vi "Login-Window.vi"(8 "Error in":errorcluster caption="Error in (no error)", 11 "Options":T1={"HideMain(T)"=TRUE, "RetryAllowed(T)"=TRUE, "LastUserToINI(T)"=TRUE}) -> (0 "Error out":errorcluster={"status"=TRUE, "code"=43, "source"="Operation cancelled by user."}, 1 "Valid User":bool, 3 "User Info":T3={"UserName"="", "Password"="", "Role"=enum."Admin"})   [LabVIEW 2017, in "Login-UI.lvlib"]
uses:
  Login-UI.lvlib
  _Typedef/Login-Account.ctl
  _Typedef/Login-Password.ctl
  _Typedef/Login-Admin.ctl
  _Typedef/Login-Confirm.ctl
  _Typedef/User-Info.ctl
  _Typedef/User-Role.ctl
  _Support/_password_db_oper.ctl
  82dbac5f-f66d-497b-81a9-0f95a8baf484.vi
  <resource>/dialog/lvconfig.llb/LV Config Read String.vi
  <resource>/dialog/lvconfig.llb/LV Config Write String.vi
panel:
  in  "UserManage":T2
  in  "Login":T5
  in  "Password":T6
  in  "UserName":T7
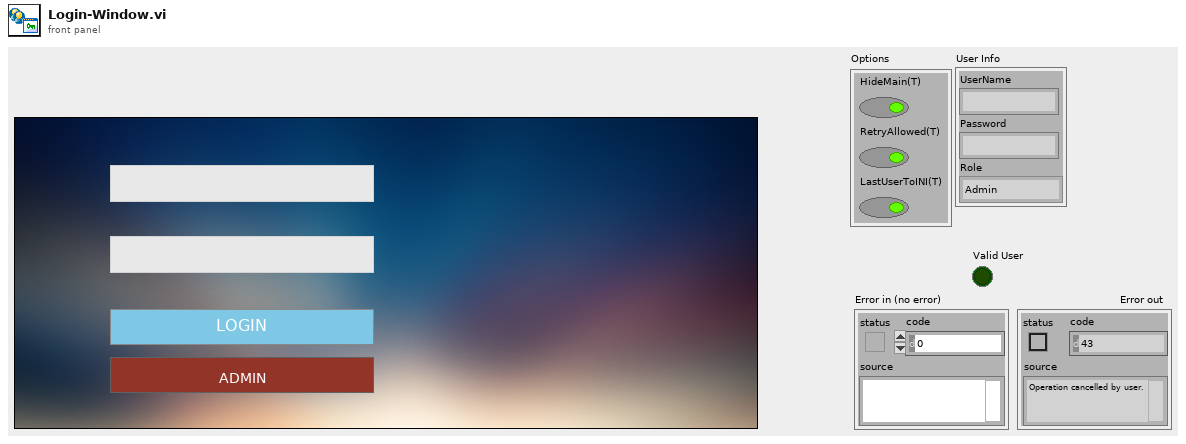
[diagram p1: front panel]
types:
  T1 = cluster{"HideMain(T)":bool, "RetryAllowed(T)":bool, "LastUserToINI(T)":bool}
  T2 = typedef "Login-UI.lvlib/Login-Admin.ctl" = bool
  T3 = typedef "Login-UI.lvlib/User-Info.ctl" = cluster{"UserName":string, "Password":string, "Role":T4}
  T4 = typedef "Login-UI.lvlib/User-Role.ctl" = enum16{"INVALID", "Operator", "Engineer", "Admin"}
  T5 = typedef "Login-UI.lvlib/Login-Confirm.ctl" = bool
  T6 = typedef "Login-UI.lvlib/Login-Password.ctl" = string
  T7 = typedef "Login-UI.lvlib/Login-Account.ctl" = string
  T8 = enum32{"Invalid", "Standard", "Closed", "Hidden", "Minimized", "Maximized"}
  T9 = typedef "Login-UI.lvlib/_password_db_oper.ctl" = enum16{"Validate", "Register", "Unregister", "View"}
  T10 = typedef "eventvkey.ctl" = enum16{"ASCII", "Enter", "Return", "Shift", "Ctrl", "Alt", "Cmd", "Opt", "Caps", "NumLock", "Clear", "Break", "Up", "Down", "Left", "Right", "Insert", "Delete", "Home", "End", "PageUp", "PageDown", "Escape", "Help", "Pause", "ScrollLock", "F1", "F2", "F3", "F4", "F5", "F6", "F7", "F8", "F9", "F10", "F11", "F12", "F13", "F14", "F15", "F16", "F17", "F18", "F19", "F20", "F21", "F22", "F23", "F24", "Play", "VolumeUp", "VolumeDown", "Mute", "Two Byte Char"}
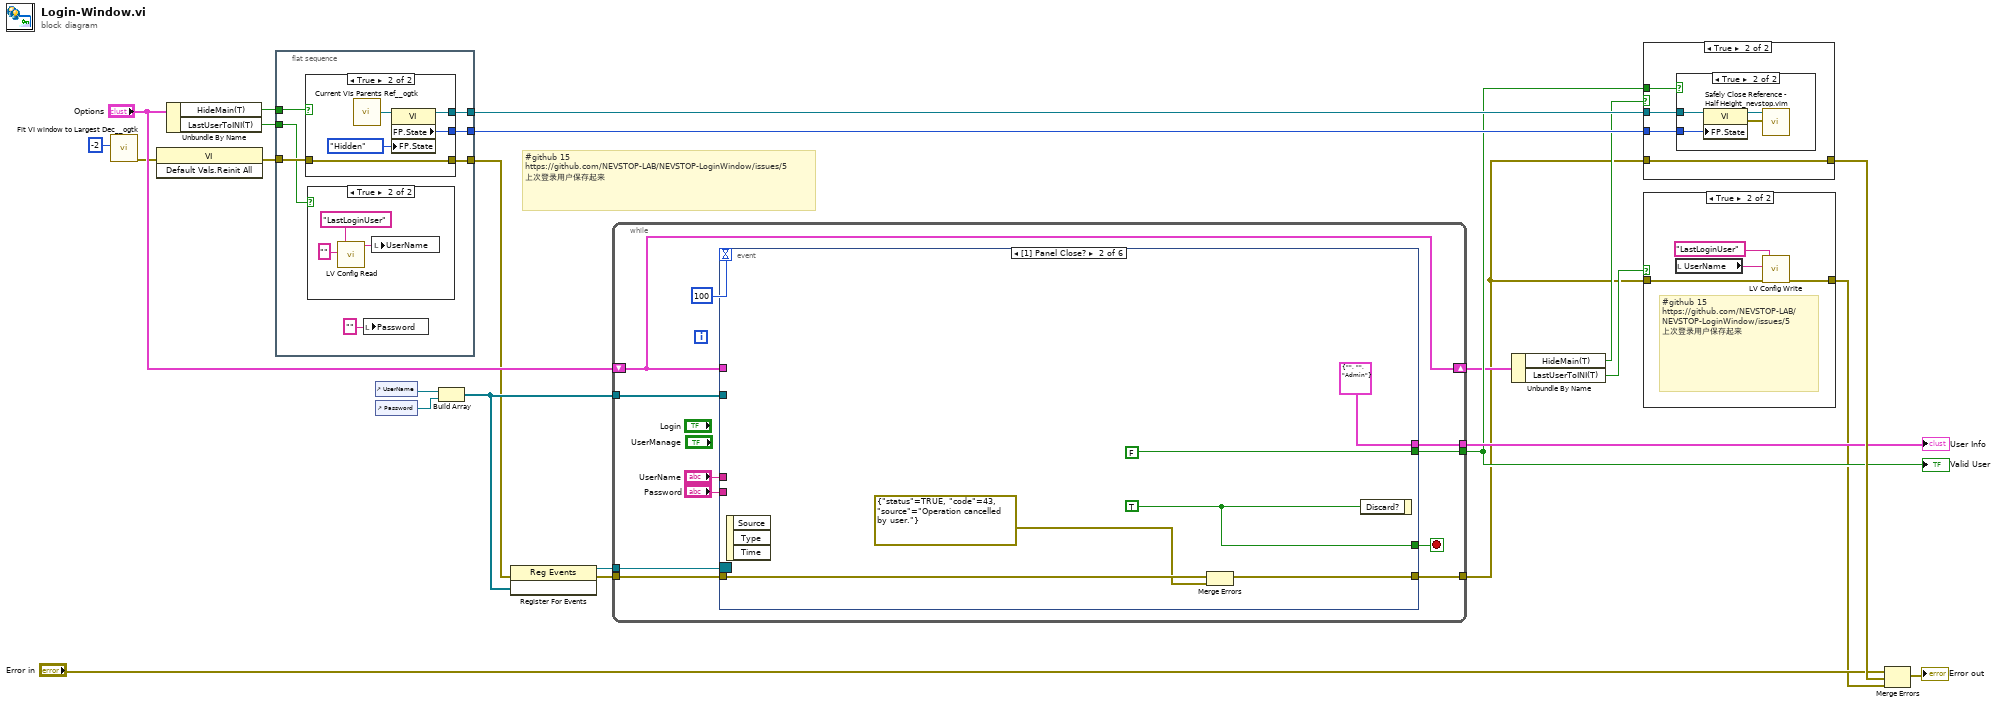
[diagram p0: block diagram]
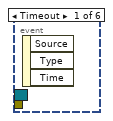
[diagram p7: hidden frame]
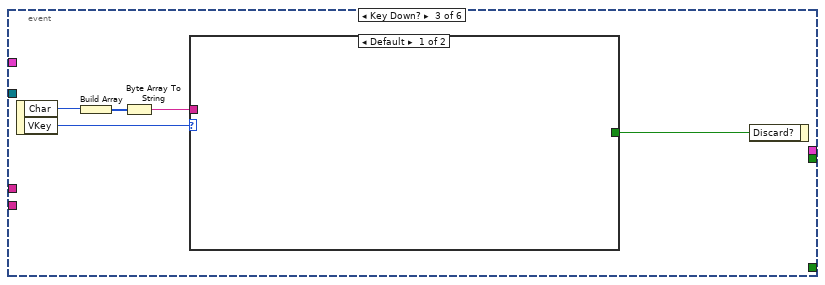
[diagram p8: hidden frame]
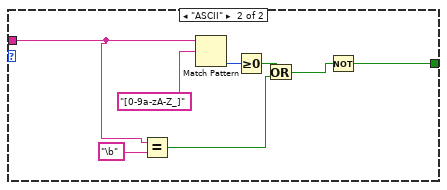
[diagram p9: hidden frame]
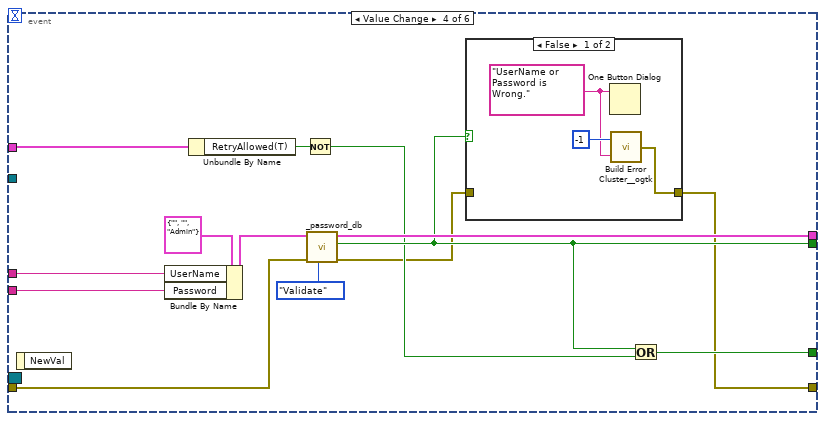
[diagram p10: hidden frame]
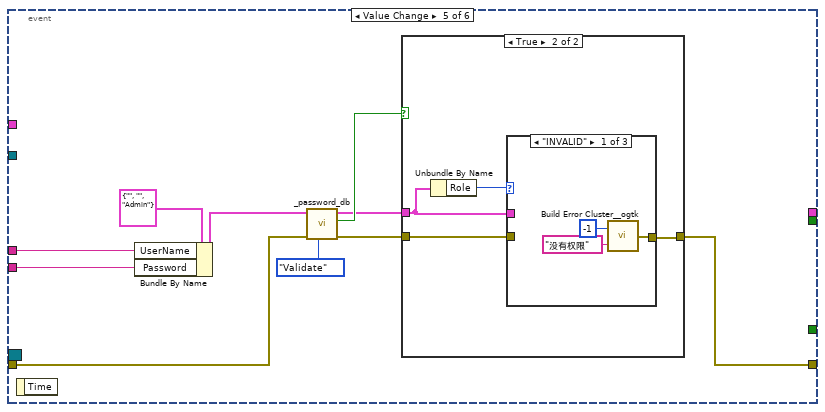
[diagram p12: hidden frame]
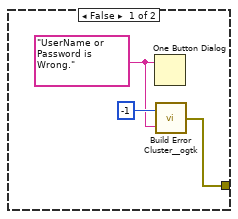
[diagram p13: hidden frame]
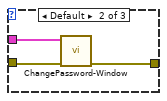
[diagram p14: hidden frame]
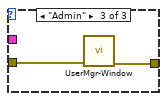
[diagram p15: hidden frame]
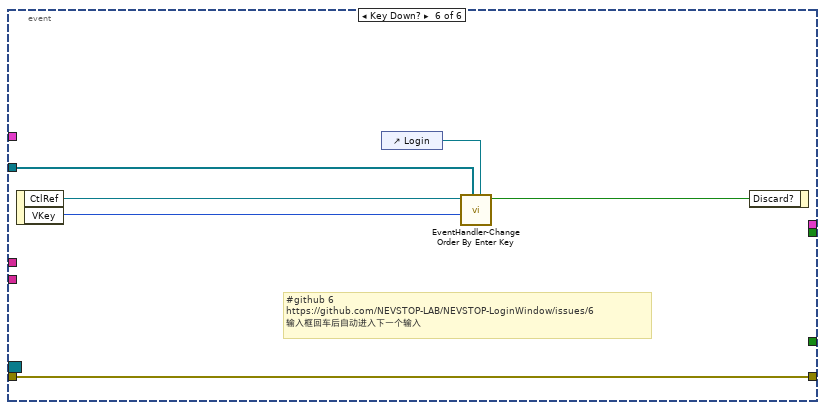
[diagram p16: hidden frame]
diagram:
  # "#github 15\nhttps://github.com/NEVSTOP-LAB/NEVSTOP-LoginWindow/issues/5\n上次登录用户保存起来"
  n1 = call <userlib>:"Fit VI window to Largest Dec__ogtk.vi"("border spacing (2 px)"=-2) -> ("error out"=w9:errorcluster)  [unwired: 5 in, 1 out]
  n2 = invoke class="VI" method="Default Vals.Reinit All"(error in=w9) -> (error out=w7:errorcluster)  [unwired: 2 in, 2 out]
  n3 = Unbundle By Name("Options") -> ("HideMain(T)"=w21:bool, "LastUserToINI(T)"=w6:bool)
  n4 = flat-sequence {
    tunnel: [w31] -> w24
    tunnel: [w30] -> w23
    tunnel: w21 -> [w29]
    tunnel: [w28] -> w8
    tunnel: w7 -> [w27]
    tunnel: w6 -> [w25]
    frame #0 {
      n5 = case shown="True" w29 {
        tunnel: [_ w38] -> w31
        tunnel: [_ w37] -> w30
        tunnel: [w35 w36] -> w28
        tunnel: w27 -> [w35 w36]
        frame False {
        }
        frame True {
          n6 = call <userlib>:"Current VIs Parents Ref__ogtk.vi"() -> ("Calling VI's Reference"=w40:refnum<vi>)  [unwired: 2 in]
          n7 = property class="VI"(reference=w40, "FP.State"=T8."Hidden" ("Front Panel Window:State")) -> (reference out=w37:refnum<vi>, "FP.State"=w38:T8)  [unwired: 1 in, 1 out]
        }
      }
      n8 = case shown="True" w25 {
        frame False {
        }
        frame True {
          n9 = call-poly <resource>:"LV Config Read.vi"("default value"="", "key"="LastLoginUser") -> ("value"=w34:string)  [unwired: 3 in, 2 out]
          n10 = local write "UserName"(w34) -> ()
        }
      }
      n11 = local write "Password"("" ("Password")) -> ()
    }
  }
  n12 = control-ref of="UserName"() -> (w15:refnum<vi>)
  n13 = control-ref of="Password"() -> (w14:refnum<vi>)
  n14 = Build Array(w15, w14) -> (w12:refnum<vi>[])
  n15 = register-events(error in=w8, w12) -> (reference out=w13:refnum<event-registration>, error out=w16:errorcluster)  [unwired: 1 in]
  n16 = while {
    tunnel: w16 -> [w47]
    tunnel: [w49] -> w20
    tunnel: [w48] -> w2
    tunnel: [w46] -> w19
    tunnel: w13 -> [w43]
    tunnel: w12 -> [w42]
    shift-right: [w41] -> w5
    shift-left: "Options" -> [w41]
    stop <- w51 stop-if-true
    n17 = event shown="[1] Panel Close?" {
      selector: w43 -> [_ _ _ _ _ _]
      dyn-events: _ -> [_ _ _ _ _ _]
      timeout: 100 -> [_ _ _ _ _ _]
      tunnel: [_ w57 _ w76 _ _] -> w51
      tunnel: [_ T3 {"UserName"="", "Password"="", "Role"=enum."Admin"} ("User Info") _ w83 _ _] -> w49
      tunnel: [_ w53 _ w73 w92 w119] -> w48
      tunnel: w47 -> [_ w55 _ w82 w97 w119]
      tunnel: [_ FALSE ("Discard?") _ w79 _ _] -> w46
      tunnel: w41 -> [_ _ _ w78 _ _]
      tunnel: "Password" -> [_ _ _ w72 w90 _]
      tunnel: "UserName" -> [_ _ _ w71 w91 _]
      tunnel: w42 -> [_ _ _ _ _ w115]
      event Timeout {
        n18 = event-data() -> ()  [unwired: 1 in, 3 out]
      }
      event Panel Close? {
        w57 = TRUE ("Discard?")
        n19 = event-data() -> ()  [unwired: 1 in, 3 out]
        n20 = Merge Errors(w55, errorcluster {"status"=TRUE, "code"=43, "source"="Operation cancelled by user."} ("error in")) -> (w53:errorcluster)
        n21 = event-data("Discard?"=w57) -> ()  [unwired: 1 in, 1 out]
      }
      event Key Down? {
        n22 = event-data() -> ("Char"=w59:i16, "VKey"=w61:T10)  [unwired: 1 in]
        n23 = Build Array(w59) -> (w60:i16[])
        n24 = Byte Array To String(unsigned byte array=w60) -> (string=w58:string)
        n25 = case shown="Default" w61 {
          tunnel: [_ w63] -> w62
          tunnel: w58 -> [_ w66]
          frame Default {
          }
          frame "ASCII" {
            n26 = Equal?(x=w66, y="\b" ("regular expression")) -> (x = y?=w64:bool)
            n27 = Match Pattern(string=w66, regular expression="[0-9a-zA-Z_]") -> (offset past match=w69:i32)  [unwired: 1 in, 3 out]
            n28 = Greater Or Equal To 0?(x=w69) -> (x >= 0?=w68:bool)
            n29 = Or(x=w68, y=w64) -> (x .or. y?=w65:bool)
            n30 = Not(x=w65) -> (.not. x?=w63:bool)
          }
        }
        n31 = event-data("Discard?"=w62) -> ()  [unwired: 1 in, 1 out]
      }
      event Value Change {
        n32 = event-data() -> ()  [unwired: 1 in, 1 out]
        n33 = Bundle By Name(cluster=T3 {"UserName"="", "Password"="", "Role"=enum."Admin"} ("Userinfo"), "UserName"=w71, "Password"=w72) -> (w80:T3)
        n34 = Unbundle By Name(w78) -> ("RetryAllowed(T)"=w77:bool)
        n35 = Not(x=w77) -> (.not. x?=w75:bool)
        n36 = call "_password_db.vi"("Enum"=_password_db_oper."Validate", "Error in"=w82, "Userinfo"=w80) -> ("Error out"=w74:errorcluster, "Boolean"=w79:bool, "Userinfo (dup)"=w83:T3)  [unwired: 5 in, 1 out]
        n37 = case shown="False" w79 {
          tunnel: w74 -> [_ w88]
          tunnel: [w85 w88] -> w73
          frame False {
            w86 = "UserName or Password is Wrong." ("message")
            n38 = One Button Dialog(message=w86) -> ()  [unwired: 1 in, 1 out]
            n39 = call <userlib>:"Build Error Cluster__ogtk.vi"("String to Prepend to source (\"\")"=w86, "code"=-1) -> ("error out"=w85:errorcluster)
          }
          frame True {
          }
        }
        n40 = Or(x=w79, y=w75) -> (x .or. y?=w76:bool)
      }
      event Value Change {
        n41 = event-data() -> ()  [unwired: 1 in, 1 out]
        n42 = Bundle By Name(cluster=T3 {"UserName"="", "Password"="", "Role"=enum."Admin"} ("Userinfo"), "UserName"=w91, "Password"=w90) -> (w95:T3)
        n43 = call "_password_db.vi"("Enum"=_password_db_oper."Validate", "Error in"=w97, "Userinfo"=w95) -> ("Error out"=w93:errorcluster, "Boolean"=w94:bool, "Userinfo (dup)"=w89:T3)  [unwired: 5 in, 1 out]
        n44 = case shown="True" w94 {
          tunnel: w93 -> [_ w105]
          tunnel: [w99 w104] -> w92
          tunnel: w89 -> [_ w102]
          frame False {
            w100 = "UserName or Password is Wrong." ("message")
            n45 = One Button Dialog(message=w100) -> ()  [unwired: 1 in, 1 out]
            n46 = call <userlib>:"Build Error Cluster__ogtk.vi"("String to Prepend to source (\"\")"=w100, "code"=-1) -> ("error out"=w99:errorcluster)
          }
          frame True {
            n47 = Unbundle By Name(w102) -> ("Role"=w103:T4)
            n48 = case shown="\"INVALID\"" w103 {
              tunnel: w105 -> [_ w111 w113]
              tunnel: [w107 w110 w112] -> w104
              tunnel: w102 -> [_ w109 _]
              frame "INVALID" {
                n49 = call <userlib>:"Build Error Cluster__ogtk.vi"("String to Prepend to source (\"\")"="没有权限" ("String to Prepend to source (\"\")"), "code"=-1) -> ("error out"=w107:errorcluster)
              }
              frame Default {
                n50 = call "ChangePassword-Window.vi"("error in (no error)"=w111, "User Info"=w109) -> ("error out"=w110:errorcluster)  [unwired: 9 in]
              }
              frame "Admin" {
                n51 = call "UserMgr-Window.vi"("error in"=w113) -> ("error out"=w112:errorcluster)  [unwired: 10 in]
              }
            }
          }
        }
      }
      event Key Down? {
        # "#github 6\nhttps://github.com/NEVSTOP-LAB/NEVSTOP-LoginWindow/issues/6\n输入框回车后自动进入下一个输入"
        n52 = event-data() -> ("CtlRef"=w117:refnum<vi>, "VKey"=w116:T10)  [unwired: 1 in]
        n53 = control-ref of="Login"() -> (w114:refnum<vi>)
        n54 = call "EventHandler-Change Order By Enter Key.vi"("Next Ctrl"=w114, "Controls for changing order"=w115, "VKey"=w116, "Event Control"=w117) -> ("Discard?"=w118:bool)  [unwired: 7 in]
        n55 = event-data("Discard?"=w118) -> ()  [unwired: 1 in, 1 out]
      }
    }
  }
  "User Info" <- w20
  "Valid User" <- w19
  n56 = Unbundle By Name(w5) -> ("HideMain(T)"=w4:bool, "LastUserToINI(T)"=w3:bool)
  n57 = case shown="True" w4 {
    tunnel: w24 -> [_ w124]
    tunnel: w23 -> [_ w123]
    tunnel: [w120 w122] -> w22
    tunnel: w2 -> [w120 w122]
    tunnel: w19 -> [_ w121]
    frame False {
    }
    frame True {
      n58 = case shown="True" w121 {
        tunnel: w124 -> [_ w128]
        tunnel: w123 -> [_ w127]
        frame False {
        }
        frame True {
          n59 = property class="VI"(reference=w127, "FP.State"=w128) -> (reference out=w125:refnum<vi>, error out=w126:errorcluster)  [unwired: 1 in]
          n60 = call "Safely Close Reference - Half Height_nevstop.vim"("error in (no error)"=w126, "Reference"=w125) -> ()  [unwired: 9 in, 1 out]
        }
      }
    }
  }
  n61 = case shown="True" w3 {
    tunnel: w2 -> [w129 w131]
    tunnel: [w129 w130] -> w1
    frame False {
    }
    frame True {
      # "#github 15\nhttps://github.com/NEVSTOP-LAB/NEVSTOP-LoginWindow/issues/5\n上次登录用户保存起来"
      n62 = local read "UserName"() -> (w132:T7)
      n63 = call-poly <resource>:"LV Config Write.vi"("error in (no error)"=w131, "value"=w132, "key"="LastLoginUser") -> ("error out"=w130:errorcluster)  [unwired: 4 in]
    }
  }
  n64 = Merge Errors("Error in", w22, w1) -> (→"Error out":errorcluster)
